vi "Log State.vi"(8 "error in (no error)":errorcluster, 10 "state":T1=enum."Start", 11 "Dispatcher in":refnum<class "Dispatcher Thread.lvclass">) -> (0 "error out":errorcluster, 3 "Dispatcher out":refnum<class "Dispatcher Thread.lvclass">)   [LabVIEW 2017, in "DSF Core.lvlib" / "Dispatcher Thread.lvclass"]
uses:
  Dispatcher Thread.lvclass
  C:/Git/DSF/Core/Classes/Thread/Thread.lvclass
  Interface/Dispatcher/Command.ctl
  <vilib>/NI/Memory Manager/Classes/Pointer/Pointer.lvclass/Pointer.ctl
  Dispatcher Thread.lvclass/Dispatcher Thread.ctl
  Interface/Logging/Command Data.ctl
  Interface/Logging/Command.ctl
  Interface/Logging/Parameters.ctl
  Interface/Logging/Dispatcher State Parameters.ctl
  Pointers/Error/Error Pointer.lvclass
  C:/Program Files (x86)/National Instruments/LabVIEW 2017/vi.lib/NI/Memory Manager/Classes/Pointer/Pointer.lvclass
  Interface/Logging/Send Logging Command.vi
  Interface/Logging/Logging Interface.lvclass
  Interface/Dispatcher/Dispatcher Interface.lvclass
  Thread.lvclass
  <vilib>/NI/Memory Manager/Classes/Pointer/Pointer.lvclass
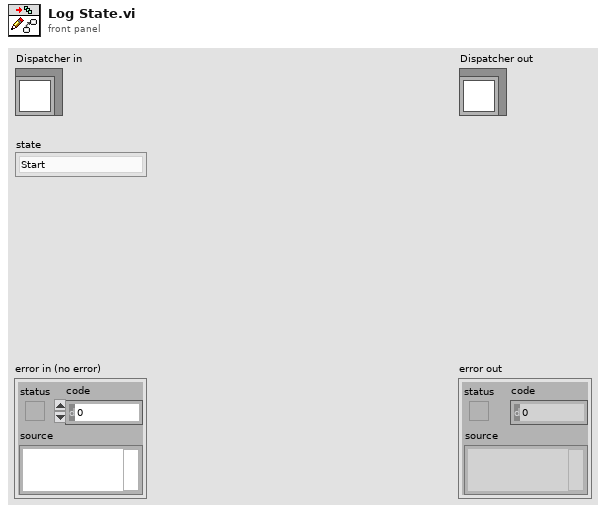
[diagram p1: front panel]
types:
  T1 = typedef "DSF Core.lvlib/Dispatcher Interface.lvclass/Command.ctl" = enum8{"Idle", "Start", "Rx", "Tx", "Set Inline Buffer", "Shutdown"}
  T2 = typedef "DSF Core.lvlib/Logging Interface.lvclass/Parameters.ctl" = cluster{"arg1":u64, "arg2":u64}
  T3 = typedef "DSF Core.lvlib/Logging Interface.lvclass/Dispatcher State Parameters.ctl" = cluster{"state":T1, "unused":u8, "unused 2":u16, "unused 3":u32, "error pointer":u64}
  T4 = typedef "DSF Core.lvlib/Logging Interface.lvclass/Command.ctl" = enum8{"Idle", "Start", "Log Framework State", "Log Plugin State", "Log Dispatcher State", "Shutdown"}
  T5 = typedef "DSF Core.lvlib/Logging Interface.lvclass/Command Data.ctl" = cluster{"Command":T4, "Parameters":T2}
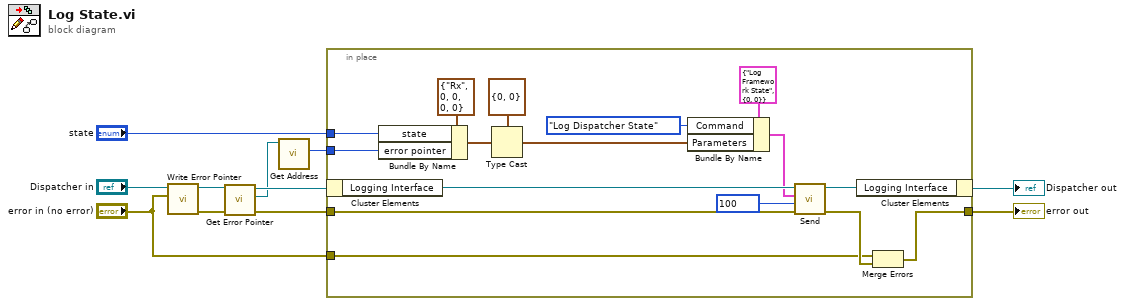
[diagram p0: block diagram]
diagram:
  n1 = call "Write Error Pointer.vi"("error"="error in (no error)", "Thread in"="Dispatcher in") -> ("error out"=w7:errorcluster, "Thread out"=w6:refnum<class "Dispatcher Thread.lvclass">)  [unwired: 8 in]
  n2 = call "Get Error Pointer.vi"("Thread in"=w6) -> ("error pointer"=w9:refnum<class "Error Pointer.lvclass">, "Thread out"=w10:refnum<class "Dispatcher Thread.lvclass">)  [unwired: 9 in]
  n3 = call <vilib>:"Get Address.vi"("Pointer in"=w9) -> ("address"=w8:u64)  [unwired: 9 in, 1 out]
  n4 = in-place {
    in-place-border: [w11] -> w3
    in-place-border: w7 -> [w21]
    in-place-border: "state" -> [w16]
    in-place-border: w8 -> [w14]
    in-place-border: "error in (no error)" -> [w12]
    n5 = in-place-cluster #1(w10) -> ("Logging Interface"=w26:refnum<class "Logging Interface.lvclass">)
    n6 = Bundle By Name(cluster=T3 {"state"=enum."Rx", "unused"=0, "unused 2"=0, "unused 3"=0, "error pointer"=0} ("Parameters"), "state"=w16, "error pointer"=w14) -> (w19:T3)
    n7 = Type Cast(type=T2 {"arg1"=0, "arg2"=0} ("Parameters"), x=w19) -> (*(type *) &x=w17:T2)
    n8 = Bundle By Name(cluster=T5 {"Command"=enum."Log Framework State", "Parameters"={"arg1"=0, "arg2"=0}} ("command"), "Command"=Command."Log Dispatcher State", "Parameters"=w17) -> (w23:T5)
    n9 = call-poly "Send.vi"("error in (no error)"=w21, "timeout in ms (0)"=100, "command"=w23, "Logging Interface in"=w26) -> ("error out"=w13:errorcluster, "Logging Interface out"=w22:refnum<class "Logging Interface.lvclass">)  [unwired: 6 in]
    n10 = in-place-cluster #1("Logging Interface"=w22) -> (→"Dispatcher out":refnum<class "Dispatcher Thread.lvclass">)
    n11 = Merge Errors(w12, w13) -> (w11:errorcluster)
  }
  "error out" <- w3
